vi "Get Thermocouple Meas Value.vi"(8 "error in (no error)":errorcluster, 11 "VISA resource name":refnum<visa-resource-name>) -> (0 "error out":errorcluster {"code" format="%.0x"}, 1 "Value Units":i32, 2 "Meas Value":dbl format="%^.3e", 3 "VISA resource name out":refnum<visa-resource-name>)   [LabVIEW 2014, in "Fluke 5XXX Series Multicalibrators.lvlib"]
doc: "This VI returns the last value of the thermocouple measurement. The unit returns indicates the status of the reading. Returns 0 and NONE when there is no recent measurement either because the Calibrator is not in a measurement mode, or because no measurement has been made yet.\n\nNote:\n\nThis VI is available only for instrument models 5500A and 5520A."
uses:
  Fluke 5XXX Series Multicalibrators.lvlib
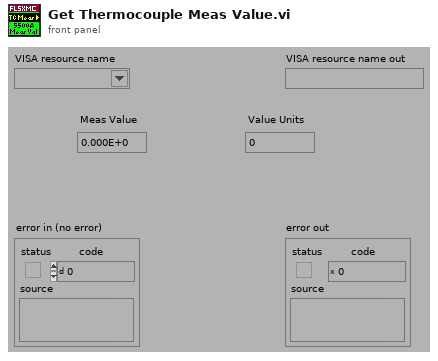
[diagram p1: front panel]
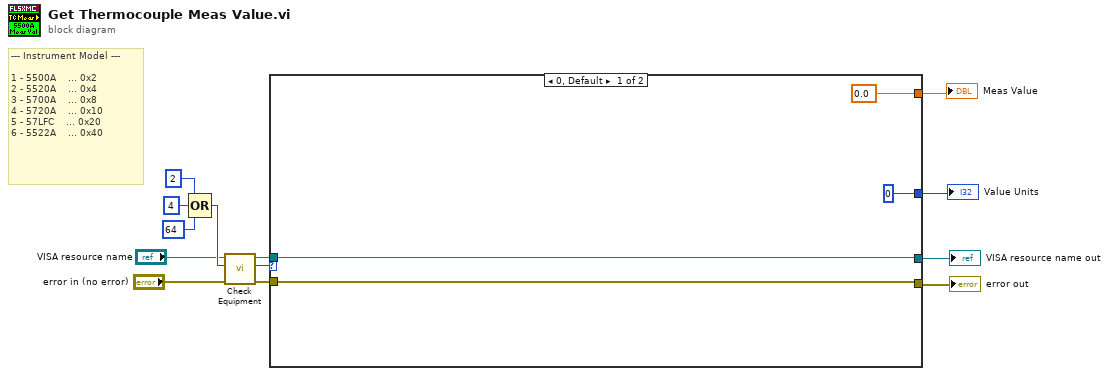
[diagram p0: block diagram]
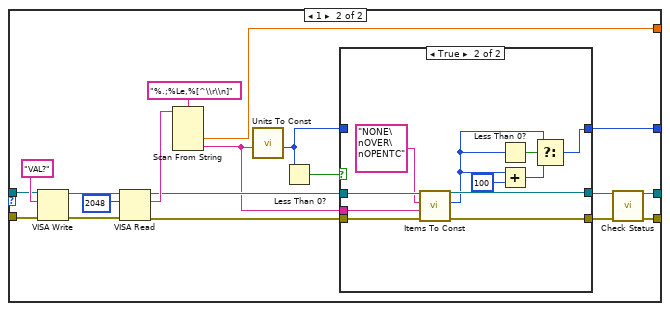
[diagram p2: hidden frame]
diagram:
  # "--- Instrument Model ---\n\n1 - 5500A    ... 0x2\n2 - 5520A    ... 0x4\n3 - 5700A    ... 0x8\n4 - 5720A    ... 0x10\n5 - 57LFC    ... 0x20\n6 - 5522A    ... 0x40"
  n1 = Compound Arithmetic op=OR(2 ("Numeric"), 4 ("Numeric"), 64 ("Numeric")) -> (w9:i32)
  n2 = call "Check Equipment.vi"("error in (no error)"="error in (no error)", "Bit Mask"=w9, "VISA resource name"="VISA resource name") -> ("error out"=w13:errorcluster, "Present?"=w12:u32, "VISA resource name out"=w2:refnum<visa-resource-name>)  [unwired: 6 in]
  n3 = case shown="0, Default" w12 {
    tunnel: [w17 w31] -> w6
    tunnel: [w14 w30] -> w5
    tunnel: w13 -> [w17 w32]
    tunnel: [0.0 w27] -> w4
    tunnel: [0 w25] -> w8
    tunnel: w2 -> [w14 w19]
    frame 0, Default {
    }
    frame 1 {
      n4 = VISA Write(VISA resource name=w19, write buffer="VAL?", error in (no error)=w32) -> (VISA resource name out=w35:refnum<visa-resource-name>, error out=w34:errorcluster)  [unwired: 1 out]
      n5 = VISA Read(VISA resource name=w35, byte count=u32 2048 ("byte count (0)"), error in (no error)=w34) -> (VISA resource name out=w24:refnum<visa-resource-name>, read buffer=w28:string, error out=w21:errorcluster)  [unwired: 1 out]
      n6 = Scan From String(format string="%.;%Le,%[^\\r\\n]", input string=w28) -> (output 1=w27:dbl, output 2=w20:string)  [unwired: 4 in, 3 out]
      n7 = call "Units To Const.vi"("Units"=w20) -> ("Const"=w18:i32)  [unwired: 10 in]
      n8 = Less Than 0?(x=w18) -> (x < 0?=w26:bool)
      n9 = case shown="True" w26 {
        tunnel: w18 -> [w39 _]
        tunnel: [w39 w46] -> w25
        tunnel: w24 -> [w37 w49]
        tunnel: [w37 w50] -> w23
        tunnel: [w38 w41] -> w22
        tunnel: w21 -> [w38 w43]
        tunnel: w20 -> [_ w47]
        frame False {
        }
        frame True {
          n10 = call "Items To Const.vi"("error in (no error)"=w43, "String Item"=w47, "Multi-Line String"="NONE\nOVER\nOPENTC", "VISA resource name"=w49) -> ("error out"=w41:errorcluster, "Index"=w40:i32, "VISA resource name out"=w50:refnum<visa-resource-name>)  [unwired: 5 in]
          n11 = Less Than 0?(x=w40) -> (x < 0?=w42:bool)
          n12 = Add(x=w40, y=100) -> (x+y=w45:i32)
          n13 = Select(t=w40, s=w42, f=w45) -> (s? t:f=w46:i32)
        }
      }
      n14 = call "Check Status.vi"("VISA resource name"=w23, "error in (no error)"=w22) -> ("VISA resource name out"=w30:refnum<visa-resource-name>, "error out"=w31:errorcluster)  [unwired: 12 in]
    }
  }
  "Meas Value" <- w4
  "Value Units" <- w8
  "VISA resource name out" <- w5
  "error out" <- w6
